vi "Tester.vi"() -> ()   [LabVIEW 2020, in "Localization_Tools.lvlib"]
uses:
  Localization_Tools.lvlib
panel:
  in  "DebugLOC":bool
  in  "Numeric 2":dbl caption="数字2"
  in  "Numeric":dbl
  in  "Array 3":bool[](array[boolean]) caption="数组3"
  in  "Array 2":dbl[](array[numeric]) caption="数组2"
  in  "Array":string[](array[string]) caption="数组"
  out "Variant":variant caption="变体"
  in  "VBAI User Palettes Folder":string="National Instruments\\Vision Builder AI\\Palettes"
  in  "VBAI Flat Field Folder":string="National Instruments\\Vision Builder AI\\Flat Field"
  in  "VBAI Calibration Folder":string="National Instruments\\Vision Builder AI\\Calibration"
  in  "Inspection Name":string="Untitled Inspection 1"
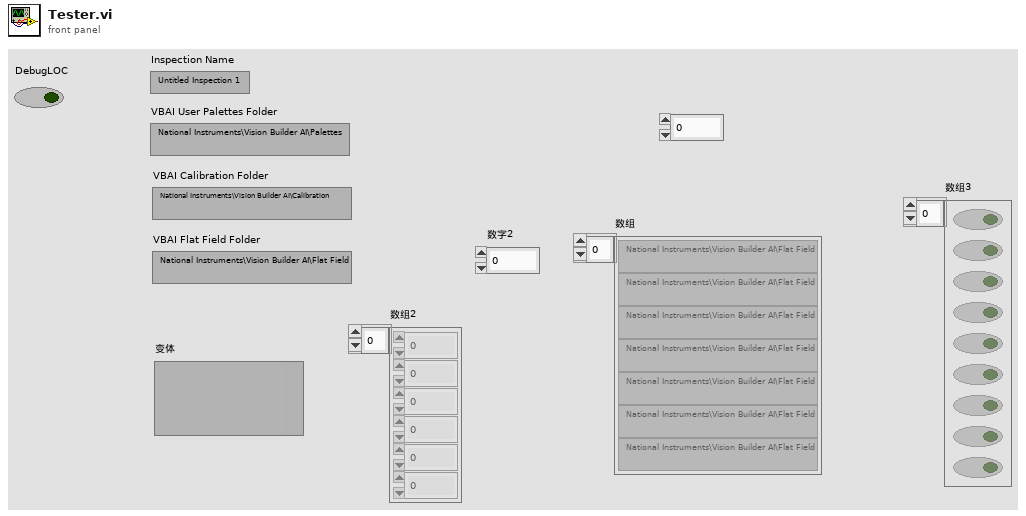
[diagram p1: front panel]
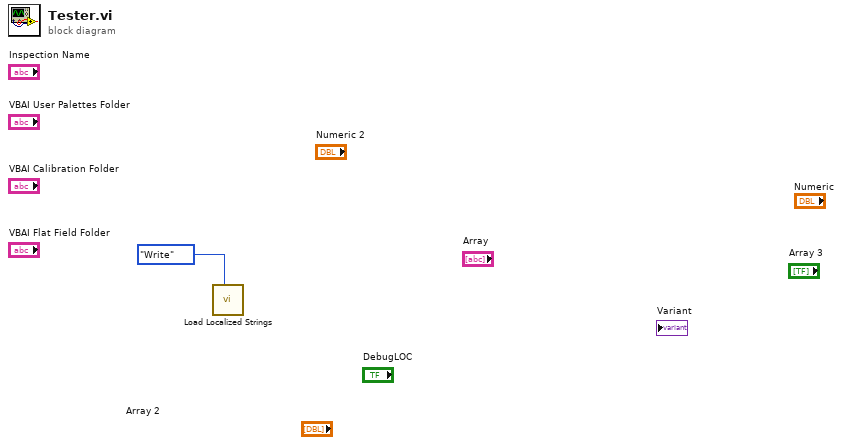
[diagram p0: block diagram]
diagram:
  n1 = call "Load Localized Strings.vi"("Mode"=enum16{"Read", "Write"}."Write") -> ()  [unwired: 9 in, 2 out]
